vi "LVPortGetTempValueMap.vi"(0 "pID":string, 5 "Object ID":i32, 7 "BaseNamepathSrc":string, 9 "Value Type (Or value to update)":variant, 11 "Object Map In":T1[](array[typedef]), 12 "BaseNamepathSrcAr":string[](array[string])) -> (4 "Object Map Out":T1[](array[typedef]))   [LabVIEW 2017]
uses:
  Common/ObjectMap/LVPortObjectMapNamepathData.ctl
  Common/ObjectMap/LVPortObjectMapDataTypeEnum.ctl
  Common/ObjectMap/LVPortObjectMapContainerTypeEnum.ctl
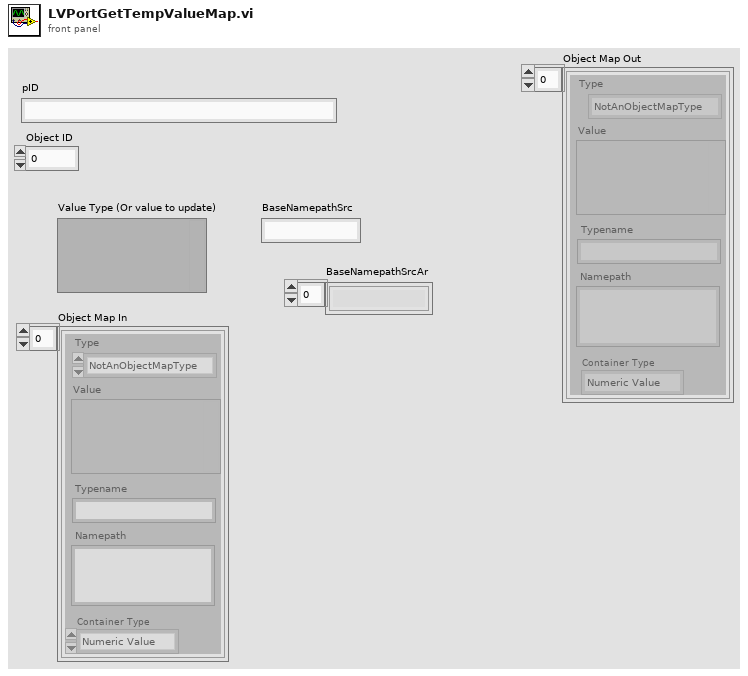
[diagram p1: front panel]
types:
  T1 = typedef "LVPortObjectMapNamepathData.ctl" = cluster{"Type":T2, "Value":variant, "Namepath":string, "Typename":string, "Container Type":T3}
  T2 = typedef "LVPortObjectMapDataTypeEnum.ctl" = enum16{"NotAnObjectMapType", "Real", "Complex", "String", "Boolean"}
  T3 = typedef "LVPortObjectMapContainerTypeEnum.ctl" = enum16{"Numeric Value", "Numeric Array", "Waveform"}
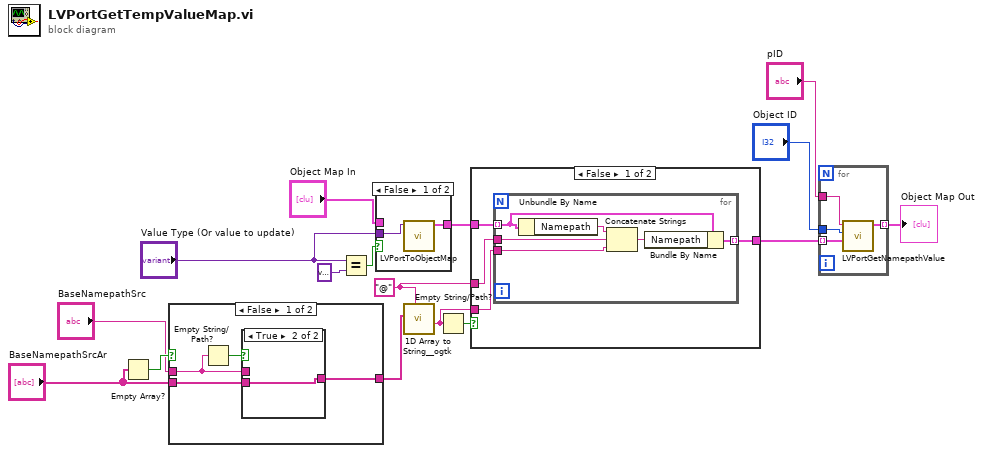
[diagram p0: block diagram]
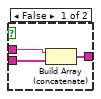
[diagram p4: hidden frame]
diagram:
  w6 = "@" ("delimiter (Tab)")
  n1 = Empty Array?(array="BaseNamepathSrcAr") -> (empty?=w16:bool)
  n2 = case shown="False" w16 {
    tunnel: "BaseNamepathSrc" -> [w20 _]
    tunnel: [w17 w25] -> w13
    tunnel: "BaseNamepathSrcAr" -> [w18 w25]
    frame False {
      n3 = Empty String/Path?(string/path=w20) -> (empty?=w19:bool)
      n4 = case shown="True" w19 {
        tunnel: w20 -> [w23 _]
        tunnel: w18 -> [w22 w24]
        tunnel: [w21 w24] -> w17
        frame False {
          n5 = Build Array (concatenate)(w23, w22) -> (w21:string[])
        }
        frame True {
        }
      }
    }
    frame True {
    }
  }
  n6 = Equal?(x="Value Type (Or value to update)", y=variant) -> (x = y?=w11:bool)
  n7 = case shown="False" w11 {
    tunnel: "Object Map In" -> [_ w28]
    tunnel: [w26 w28] -> w7
    tunnel: "Value Type (Or value to update)" -> [w27 _]
    frame False {
      n8 = call "LVPortToObjectMap.vi"("Value"=w27) -> ("Object map"=w26:T1[])  [unwired: 10 in]
    }
    frame True {
    }
  }
  n9 = call <userlib>:"1D Array to String__ogtk.vi"("delimiter (Tab)"=w6, "Array of Strings"=w13) -> ("delimited string"=w5:string)  [unwired: 9 in]
  n10 = Empty String/Path?(string/path=w5) -> (empty?=w8:bool)
  n11 = case shown="False" w8 {
    tunnel: w7 -> [w32 w39]
    tunnel: w6 -> [w31 _]
    tunnel: w5 -> [w30 _]
    tunnel: [w29 w39] -> w4
    frame False {
      n12 = for {
        tunnel: w32 -> [w38] mode=indexing
        tunnel: w31 -> [w36]
        tunnel: w30 -> [w35]
        tunnel: [w34] -> w29 mode=indexing
        n13 = Unbundle By Name(w38) -> ("Namepath"=w37:string)
        n14 = Concatenate Strings(w37, w36, w35) -> (w33:string)
        n15 = Bundle By Name(cluster=w38, "Namepath"=w33) -> (w34:T1)
      }
    }
    frame True {
    }
  }
  n16 = for {
    tunnel: w4 -> [w43] mode=indexing
    tunnel: "pID" -> [w42]
    tunnel: "Object ID" -> [w41]
    tunnel: [w40] -> w1 mode=indexing
    n17 = call "LVPortGetNamepathValue.vi"("Namepath Data in"=w43, "Object ID"=w41, "pID"=w42) -> ("Namepath Data out"=w40:T1)  [unwired: 8 in]
  }
  "Object Map Out" <- w1
